vi "client.vi"() -> ()   [LabVIEW 2019]
uses:
  Generated_client/RPC Messages/helloworld_HelloRequest.ctl
  Generated_client/RPC Messages/helloworld_HelloReply.ctl
  Generated_client/Generated_client.lvlib
panel:
  out "helloworld_HelloReply":T1
  in  "helloworld_HelloRequest":T2={"name"="Dan"}
  in  "error in (no error)":errorcluster
  out "error out":errorcluster
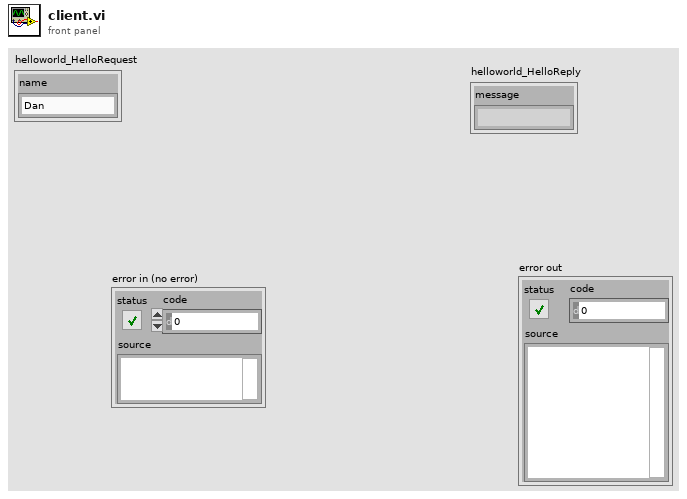
[diagram p1: front panel]
types:
  T1 = typedef "Generated_client.lvlib/helloworld_HelloReply.ctl" = cluster{"message":string}
  T2 = typedef "Generated_client.lvlib/helloworld_HelloRequest.ctl" = cluster{"name":string}
  T3 = typedef "grpc-lvsupport-release.lvlib/grpcId.ctl" = u64
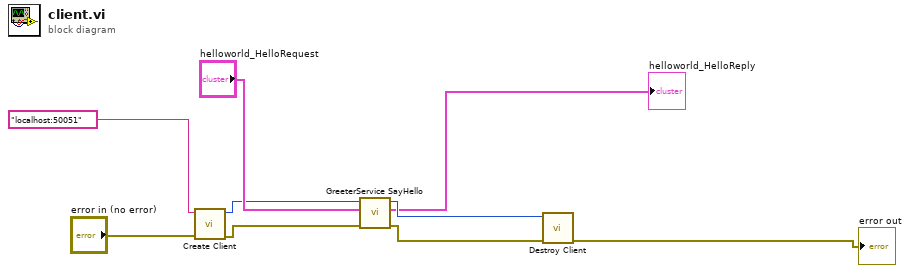
[diagram p0: block diagram]
diagram:
  n1 = call "Create Client.vi"("error in"="error in (no error)", "address"="localhost:50051") -> ("error out"=w3:errorcluster, "gRPC ID Out"=w6:T3)  [unwired: 8 in]
  n2 = call "GreeterService SayHello.vi"("error in"=w3, "Request Data"="helloworld_HelloRequest", "gRPC ID"=w6) -> ("error out"=w2:errorcluster, "Response Data"=→"helloworld_HelloReply":T1, "gRPC ID out"=w5:T3)  [unwired: 6 in]
  n3 = call "Destroy Client.vi"("error in"=w2, "gRPC ID"=w5) -> ("error out"=→"error out":errorcluster)  [unwired: 9 in]
